vi "Get Array Element.vi"(5 "Key name":string, 6 "Index":i32=4, 7 "Section name":string, 8 "error in (no error)":errorcluster, 9 "Use Key Regex? [F]":bool, 10 "Use Section Regex? [F]":bool, 11 "Carya Config in":refnum<class "Carya Config.lvclass">) -> (0 "error out":errorcluster, 1 "Key names":string[](array[string]), 2 "Section names":string[](array[string]), 3 "Carya Config out":refnum<class "Carya Config.lvclass">, 4 "Values":string[](array[string]))   [LabVIEW 2013, in "Carya Config.lvclass"]
doc: "Copyright 2018, Carya Automatisering, Wiebe Walstra."
uses:
  Carya Config.lvclass
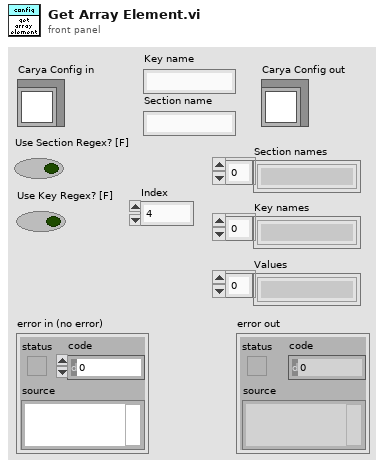
[diagram p1: front panel]
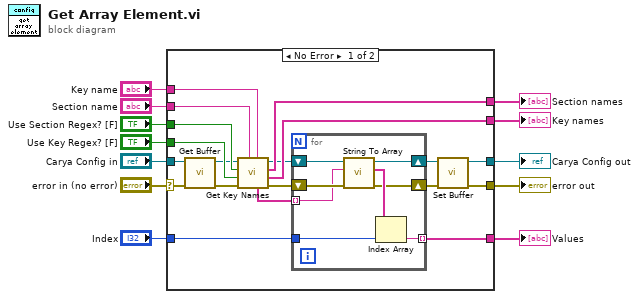
[diagram p0: block diagram]
diagram:
  n1 = case shown="No Error" "error in (no error)" {
    selector: "error in (no error)" -> [w31 w41]
    tunnel: [w30 w41] -> w11
    tunnel: [w29 w40] -> w9
    tunnel: "Carya Config in" -> [w23 w40]
    tunnel: "Section name" -> [w26 _]
    tunnel: "Key name" -> [w25 _]
    tunnel: "Use Section Regex? [F]" -> [w28 _]
    tunnel: "Use Key Regex? [F]" -> [w27 _]
    tunnel: "Index" -> [w24 _]
    tunnel: [w22 _] -> w3
    tunnel: [w21 _] -> w2
    tunnel: [w20 _] -> w1
    frame No Error {
      n2 = call-dynamic "Get Buffer.vi"("error in (no error)"=w31, "Carya Config in"=w23) -> ("error out"=w13:errorcluster, "Config"=w14:refnum<class "Carya Config.lvclass">)  [unwired: 8 in]
      n3 = call-dynamic "Get Key Names.vi"("Key name/Regex"=w25, "Section name/Regex"=w26, "error in (no error)"=w13, "Use Key Regex? [F]"=w27, "Use Section Regex? [F]"=w28, "Carya Config in"=w14) -> ("error out"=w18:errorcluster, "Key names"=w21:string[], "Section names"=w22:string[], "Carya Config out"=w16:refnum<class "Carya Config.lvclass">, "Context (concatenated)"=w19:string[])  [unwired: 1 in]
      n4 = for {
        shift-right: [w34] -> w17
        shift-left: w16 -> [w38]
        shift-right: [w33] -> w15
        shift-left: w18 -> [w39]
        tunnel: w19 -> [w37] mode=indexing
        tunnel: w24 -> [w36]
        tunnel: [w32] -> w20 mode=indexing
        n5 = call-dynamic "String To Array.vi"("error in (no error)"=w39, "resulting string"=w37, "Registry Object"=w38) -> ("error out"=w33:errorcluster, "Array"=w35:string[], "Registry Object"=w34:refnum<class "Carya Config.lvclass">)  [unwired: 6 in]
        n6 = Index Array(array=w35, index=w36) -> (element=w32:string)
      }
      n7 = call-dynamic "Set Buffer.vi"("error in (no error)"=w15, "Carya Config"=w17) -> ("error out"=w30:errorcluster, "Carya Config out"=w29:refnum<class "Carya Config.lvclass">)  [unwired: 8 in]
    }
    frame Error {
    }
  }
  "error out" <- w11
  "Carya Config out" <- w9
  "Section names" <- w3
  "Key names" <- w2
  "Values" <- w1
